vi "if VI is running stop VI.vi"(8 "error in (no error)":errorcluster, 11 "VI in":refnum<vi>) -> (0 "error out":errorcluster, 3 "VI out":refnum<vi>)   [LabVIEW 2023]
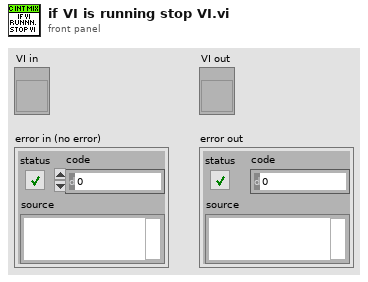
[diagram p1: front panel]
types:
  T1 = enum32{"Bad", "Idle", "Run top level", "Running"}
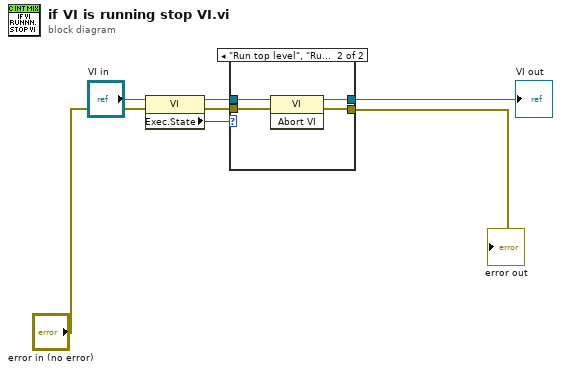
[diagram p0: block diagram]
diagram:
  n1 = property class="VI"(reference="VI in", error in="error in (no error)") -> (reference out=w5:refnum<vi>, error out=w4:errorcluster, "Exec.State"=w3:T1)
  n2 = case shown="\"Run top level\", \"Running\"" w3 {
    tunnel: w4 -> [w8 w13]
    tunnel: w5 -> [w9 w12]
    tunnel: [w9 w11] -> w6
    tunnel: [w8 w10] -> w7
    frame "Bad", Default {
    }
    frame "Run top level", "Running" {
      n3 = invoke class="VI" method="Abort VI"(reference=w12, error in=w13) -> (reference out=w11:refnum<vi>, error out=w10:errorcluster)  [unwired: 1 in, 1 out]
    }
  }
  "error out" <- w7
  "VI out" <- w6
